vi "Core Actor (ROOT) - Dispatch Message to Child (Nested_Actor).vi"(8 "error in (no error)":errorcluster, 11 "Child_2_Class in":refnum<class "Console_Class.lvclass">) -> (0 "error out":errorcluster, 3 "Child_2_Class out":refnum<class "Console_Class.lvclass">)   [LabVIEW 2023, in "Console_Actor.lvlib" / "Console_Class.lvclass"]
uses:
  Console_Class.lvclass
  Console_Class.lvclass/Console_Class.ctl
  Console_Class Messages/Core Actor - Send Actor Message Msg/Core Actor - Send Actor Message Msg.lvclass/Core Actor - Send Actor Message Msg.ctl
  <vilib>/ActorFramework/Message Enqueuer/Message Enqueuer.lvclass/Message Enqueuer.ctl
  <vilib>/ActorFramework/Message Enqueuer/Enqueue.vi
  Console_Class Messages/Core Actor - Send Actor Message Msg/Core Actor - Send Actor Message Msg.lvclass
  Applications/National Instruments/LabVIEW 2023 64-bit/vi.lib/ActorFramework/Message/Message.lvclass
  <vilib>/ActorFramework/Message Priority Queue/Priority Enqueue.vi
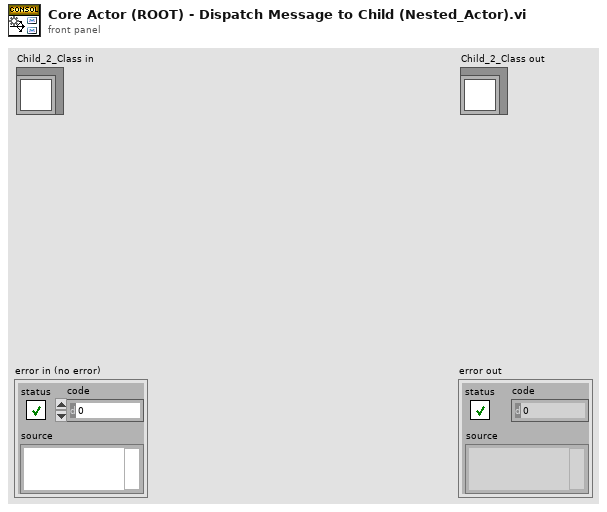
[diagram p1: front panel]
types:
  T1 = typedef "Console_Actor.lvlib/Console_Class.lvclass/Child 2 - Ctrl - Trigger Event Cluster.ctl" = cluster{"Events":T2, "Data":string}
  T2 = typedef "Console_Actor.lvlib/Console_Class.lvclass/Child_2 - Ctrl - Enum - Events (Temp).ctl" = enum16{"SEND MESSAGE Ev", "STOP_ACTOR Ev", "INIT_ACTOR Ev", "START Ev", "STOP Ev", "GET Ev", "SET Ev", "ERROR_HANDLER Ev", "RESET Ev", "T2 Ev", "T3 Ev", "T4 Ev"}
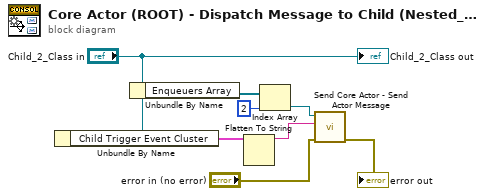
[diagram p0: block diagram]
diagram:
  n1 = Unbundle By Name("Child_2_Class in") -> ("Child Trigger Event Cluster"=w2:T1)
  n2 = Unbundle By Name("Child_2_Class in") -> ("Enqueuers Array"=w8:refnum<class "Message Enqueuer.lvclass">[])
  n3 = Flatten To String(anything=w2) -> (data string=w1:string)  [unwired: 3 in, 2 out]
  n4 = Index Array(array=w8, index=2) -> (element=w6:refnum<class "Message Enqueuer.lvclass">)
  n5 = call "Send Core Actor - Send Actor Message.vi"("error in (no error)"="error in (no error)", "Value"=w1, "Message Enqueuer"=w6) -> ("error out"=→"error out":errorcluster)  [unwired: 7 in, 1 out]
  "Child_2_Class out" <- "Child_2_Class in"
